vi "Write.vi"(8 "error in (no error)":errorcluster, 10 "MeasurementData":T1, 11 "TXT_Writer in":refnum<class "TXT_Writer.lvclass">) -> (0 "error out":errorcluster, 3 "TXT_Writer out":refnum<class "TXT_Writer.lvclass">)   [LabVIEW 2024, in "Data.lvlib" / "TXT_Writer.lvclass"]
uses:
  TXT_Writer.lvclass
  C:/Users/aheme/Documents/Dev/DEV_INFO/DEV_INFO/StockM/MyLabVIEW_Framework/Data/DataWriter/DataWriter.lvclass
  Data/DataModel/MeasurementData.ctl
  Controls/SensorType.ctl
  Controls/Config.ctl
  Data/DataWriter/DataWriter.lvclass/DataWriter.ctl
  Data/DataWriter/DataWriter.lvclass
  Sensors.lvlib
  Data.lvlib
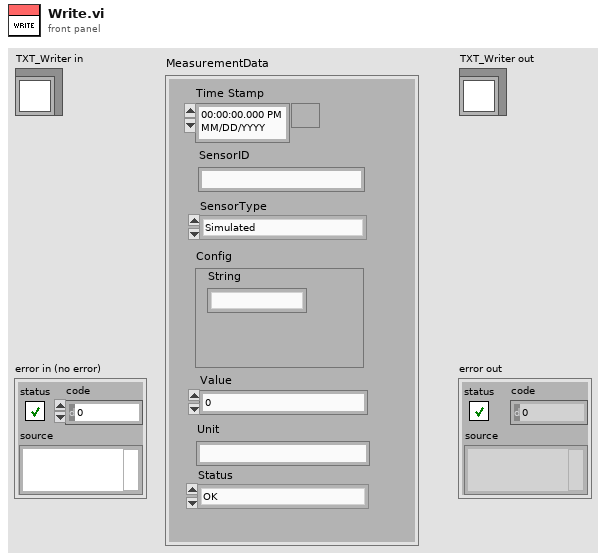
[diagram p1: front panel]
types:
  T1 = typedef "Data.lvlib/MeasurementData.ctl" = cluster{"Time Stamp":timestamp, "SensorID":string, "SensorType":T2, "Config":T3, "Value":dbl, "Unit":string, "Status":enum16{"OK", "Warning", "Error"}}
  T2 = typedef "Sensors.lvlib/SensorType.ctl" = enum16{"Simulated", "pH", "NPK"}
  T3 = typedef "Sensors.lvlib/Config.ctl" = cluster{"String":string}
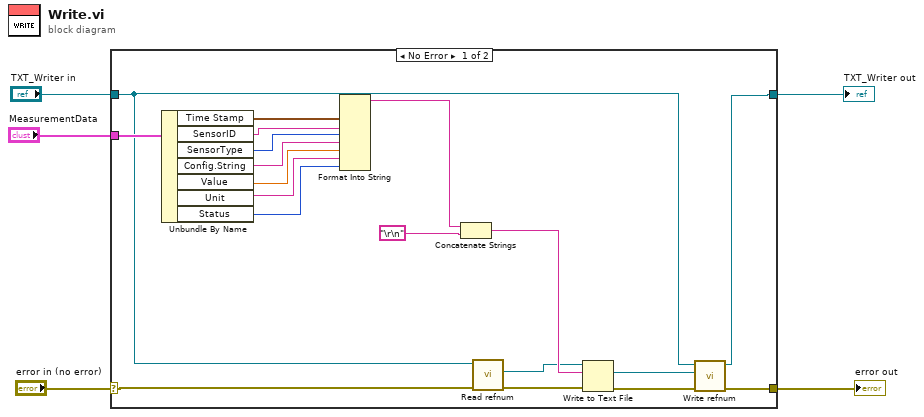
[diagram p0: block diagram]
diagram:
  n1 = case shown="No Error" "error in (no error)" {
    selector: "error in (no error)" -> [w7 w26]
    tunnel: [w23 w26] -> w5
    tunnel: [w21 w25] -> w4
    tunnel: "TXT_Writer in" -> [w8 w25]
    tunnel: "MeasurementData" -> [w20 _]
    frame No Error {
      n2 = Unbundle By Name(w20) -> ("Time Stamp"=w19:timestamp, "SensorID"=w17:string, "SensorType"=w18:T2, "Config.String"=w16:string, "Value"=w15:dbl, "Unit"=w14:string, "Status"=w13:enum16{"OK", "Warning", "Error"})
      n3 = Format Into String(w19, w17, w18, w16, w15, w14, w13) -> (resulting string=w12:string)  [unwired: 3 in, 1 out]
      n4 = Concatenate Strings(w12, "\r\n") -> (w10:string)
      n5 = call "Read refnum.vi"("error in (no error)"=w7, "DataWriter in"=w8) -> ("error out"=w6:errorcluster, "refnum"=w9:refnum<file>)  [unwired: 7 in, 1 out]
      n6 = Write to Text File(file (use dialog)=w9, text=w10, error in=w6) -> (refnum out=w22:refnum<file>, error out=w24:errorcluster)  [unwired: 1 in, 1 out]
      n7 = call "Write refnum.vi"("error in (no error)"=w24, "refnum"=w22, "DataWriter in"=w8) -> ("error out"=w23:errorcluster, "DataWriter out"=w21:refnum<class "TXT_Writer.lvclass">)  [unwired: 7 in]
    }
    frame Error {
    }
  }
  "error out" <- w5
  "TXT_Writer out" <- w4
